vi "Close.vi"(8 "error in":errorcluster, 11 "IClose in":refnum<class "IClose.lvclass">) -> (0 "error out":errorcluster, 3 "IClose out":refnum<class "IClose.lvclass">)   [LabVIEW 2024, in "IClose.lvclass"]
uses:
  IClose.lvclass
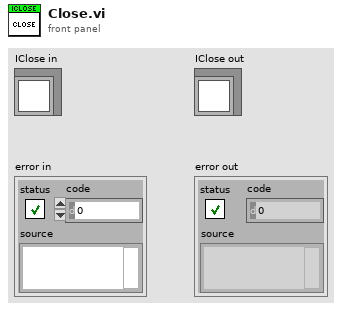
[diagram p1: front panel]
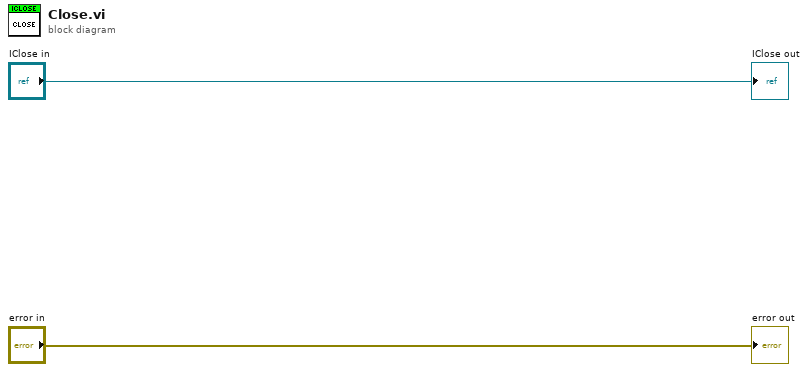
[diagram p0: block diagram]
diagram:
  "error out" <- "error in"
  "IClose out" <- "IClose in"
